vi "Inclinometer_Scale_Units.vi"(5 "Enum":T1=enum."Azim", 7 "Inclin":T2, 11 "Unscaled":dbl) -> (3 "Scaled":dbl)   [LabVIEW 2018]
doc: "Angle_out = ((Voltage_reading / 4.5) * 180) - 90\n \nwhere: \n-\"Angle_out\" is the angle reading we are interested in (in degrees)\n-\"Voltage_reading\" is the voltage at the NI input terminal (in volts)\n-\"4.5\" is the maximum voltage output of the device (in volts)\n-\"180\" is the angle range (in degrees)\n-\"90\" is the offset due to having a positive and negative angle range (voltage reading of 2.25 V translates to 0 degrees)\n \nThere may be a desire to change the output settings, so the following generic formula may be more appropriate to implement:\n \nAngle_out = ((Voltage_reading / Voltage_max) * Angle_range) - (Angle_range / 2)\n \nwhere \"Angle_range\" and \"Voltage_max\" require user input to define and the range is assumed to be symmetric about zero.\n\nFrom Jordan Keeley, 16 May 2019"
uses:
  Controls/Clusts/Inclinometer_User_Cfg.ctl
  Controls/Enums/Inclinometer_Direction.ctl
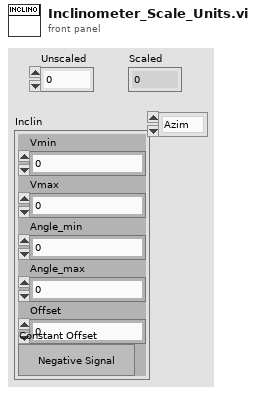
[diagram p1: front panel]
types:
  T1 = typedef "Inclinometer_Direction.ctl" = enum16{"Elev", "Azim"}
  T2 = typedef "Inclinometer_User_Cfg.ctl" = cluster{"Vmin":dbl, "Vmax":dbl, "Angle_min":dbl, "Angle_max":dbl, "Offset":dbl, "Pos_Neg":bool}
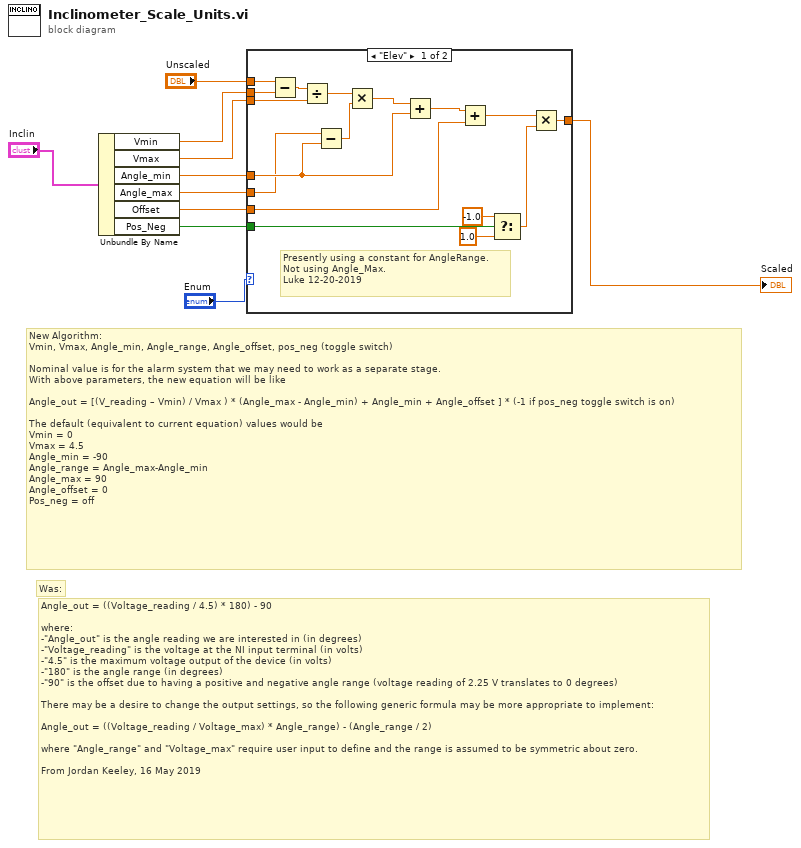
[diagram p0: block diagram]
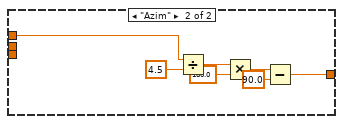
[diagram p2: hidden frame]
diagram:
  # "New Algorithm:\nVmin, Vmax, Angle_min, Angle_range, Angle_offset, pos_neg (toggle switch)\n\nNominal value is for the alarm system that we may need to work as a separate stage.\nWith above parameters, the new equation will be like\n\nAngle_out = [(V_reading – Vmin) / Vmax ) * (Angle_max - Angle_min) + Angle_min + Angle_offset ] * (-1 if pos_neg toggle switch is on)\n\nThe default (equivalent to current equation) values would be\nVmin = 0\nVmax = 4.5\nAngle_min = -90\nAngle_range = Angle_max-Angle_min\nAngle_max = 90\nAngle_offset = 0\nPos_neg = off"
  # "Was:"
  # "Angle_out = ((Voltage_reading / 4.5) * 180) - 90\n \nwhere: \n-\"Angle_out\" is the angle reading we are interested in (in degrees)\n-\"Voltage_reading\" is the voltage at the NI input terminal (in volts)\n-\"4.5\" is the maximum voltage output of the device (in volts)\n-\"180\" is the angle range (in degrees)\n-\"90\" is the offset due to having a positive and negative angle range (voltage reading of 2.25 V translates to 0 degrees)\n \nThere may be a desire to change the output settings, so the following generic formula may be more appropriate to implement:\n \nAngle_out = ((Voltage_reading / Voltage_max) * Angle_range) - (Angle_range / 2)\n \nwhere \"Angle_range\" and \"Voltage_max\" require user input to define and the range is assumed to be symmetric about zero.\n\nFrom Jordan Keeley, 16 May 2019"
  n1 = Unbundle By Name("Inclin") -> ("Vmin"=w7:dbl, "Vmax"=w6:dbl, "Angle_min"=w5:dbl, "Angle_max"=w2:dbl, "Offset"=w4:dbl, "Pos_Neg"=w3:bool)
  n2 = case shown="\"Elev\"" "Enum" {
    tunnel: [w27 w28] -> w10
    tunnel: "Unscaled" -> [w26 w29]
    tunnel: w7 -> [w25 _]
    tunnel: w6 -> [w24 _]
    tunnel: w5 -> [w23 _]
    tunnel: w4 -> [w22 _]
    tunnel: w3 -> [w21 _]
    tunnel: w2 -> [w20 _]
    frame "Elev" {
      # "Presently using a constant for AngleRange.\nNot using Angle_Max.\nLuke 12-20-2019"
      n3 = Subtract(x=w26, y=w25) -> (x-y=w19:dbl)
      n4 = Divide(x=w19, y=w24) -> (x/y=w18:dbl)
      n5 = Subtract(x=w20, y=w23) -> (x-y=w11:dbl)
      n6 = Multiply(x=w18, y=w11) -> (x*y=w17:dbl)
      n7 = Add(x=w17, y=w23) -> (x+y=w16:dbl)
      n8 = Add(x=w16, y=w22) -> (x+y=w15:dbl)
      n9 = Select(t=-1.0, s=w21, f=1.0) -> (s? t:f=w14:dbl)
      n10 = Multiply(x=w15, y=w14) -> (x*y=w27:dbl)
    }
    frame "Azim" {
      n11 = Divide(x=w29, y=4.5) -> (x/y=w33:dbl)
      n12 = Multiply(x=w33, y=180.0) -> (x*y=w34:dbl)
      n13 = Subtract(x=w34, y=90.0) -> (x-y=w28:dbl)
    }
  }
  "Scaled" <- w10
